vi "Clear board.vi"(11 "Board in":refnum<class "Board.lvclass">) -> (3 "Board out":refnum<class "Board.lvclass">)   [LabVIEW 2015, in "Chesslib.lvlib" / "Board.lvclass"]
uses:
  Board.lvclass
  Board.lvclass/Board.ctl
  Pieces/Piece/Piece.lvclass
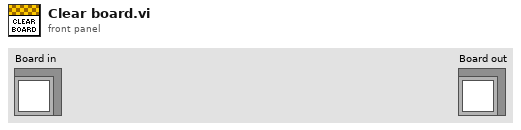
[diagram p1: front panel]
types:
  T1 = cluster{"Occupied":bool, "Piece":refnum<class "Piece.lvclass">}[]
  T2 = cluster{"Occupied":bool, "Piece":refnum<class "Piece.lvclass">}
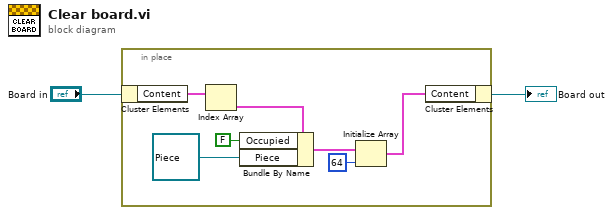
[diagram p0: block diagram]
diagram:
  n1 = in-place "In Place Element Structure" {
    n2 = in-place-cluster #1("Board in") -> ("Content"=w7:T1)
    n3 = Index Array(array=w7) -> (element=w6:T2)  [unwired: 1 in]
    n4 = Bundle By Name(cluster=w6, "Occupied"=FALSE, "Piece"=refnum<class "Piece.lvclass"> refnum) -> (w3:T2)
    n5 = Initialize Array(w3, 64 ("dimension size")) -> (w9:T1)
    n6 = in-place-cluster #1("Content"=w9) -> (→"Board out":refnum<class "Board.lvclass">)
  }
